vi "Notifier.vi"() -> ()   [LabVIEW 2021]
panel:
  out "Numeric 2":i32
  out "Numeric":i32
  in  "stop":bool
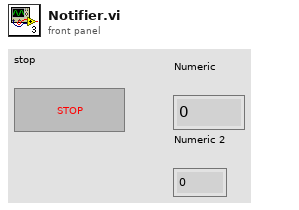
[diagram p1: front panel]
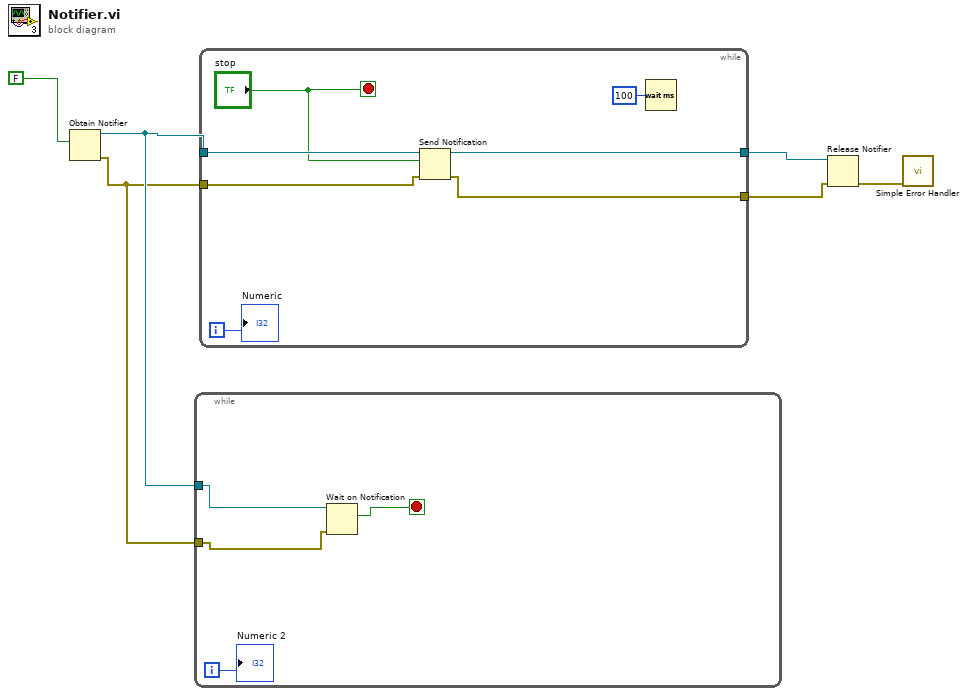
[diagram p0: block diagram]
diagram:
  n1 = Obtain Notifier(notification data type=FALSE) -> (notifier out=w2:refnum<notifier>, error out=w1:errorcluster)  [unwired: 3 in, 1 out]
  n2 = while {
    tunnel: w2 -> [w10]
    tunnel: w1 -> [w9]
    i -> [w7]
    stop <- w8 stop-if-true
    n3 = Wait on Notification(notifier=w10, error in (no error)=w9) -> (notification=w8:bool)  [unwired: 2 in, 3 out]
    "Numeric 2" <- w7
  }
  n4 = while {
    tunnel: w2 -> [w17]
    tunnel: w1 -> [w16]
    tunnel: [w15] -> w5
    tunnel: [w14] -> w4
    i -> [w11]
    stop <- "stop" stop-if-true
    n5 = Send Notification(notification="stop", notifier=w17, error in (no error)=w16) -> (notifier out=w15:refnum<notifier>, error out=w14:errorcluster)
    n6 = Wait (ms)(milliseconds to wait=u32 100) -> ()  [unwired: 1 out]
    "Numeric" <- w11
  }
  n7 = Release Notifier(notifier=w5, error in (no error)=w4) -> (error out=w3:errorcluster)  [unwired: 1 in, 2 out]
  n8 = call <vilib>:"Simple Error Handler.vi"("error in (no error)"=w3) -> ()  [unwired: 4 in, 5 out]
